vi "DjtgPutTmsTdiBits.vi"(6 "Receive Buffer Size (Bytes)":i32=10, 7 "Overlap?":bool, 8 "Error In":errorcluster, 9 "Num Bit Pairs":u32, 10 "Data To Send":u8[](array[numeric]), 11 "Device Number":u32) -> (0 "Error Out":errorcluster, 2 "Data":u8[](array[numeric]), 3 "Device Number":u32)   [LabVIEW 2011, in "LVH-Adept.lvlib" / "DJTG.lvlib"]
doc: "Regardless of the scan format configuration, the rgbSnd parameter specifies a buffer containing the sequence of the TDI and TMS bits that should be shifted. The TDI bits contained in rgbSnd are automatically complemented as necessary. For example, if the current scan format is OScan1 and rgbSnd[0] = 0xAB and rgbSnd[1] = 0xEB then first byte of TDI bits is 0x91 and 0x6E will be shifted for the nTDI bits. For more information regarding the format of the data shifted by this function, see the section titled “Scan Formats.”"
uses:
  DJTG.lvlib
  Private/Type Defs/Error.ctl
  Resources/djtg.dll
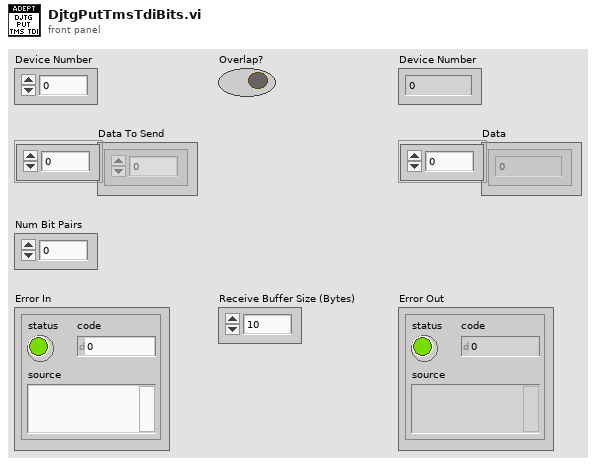
[diagram p1: front panel]
types:
  T1 = typedef "LVH-Adept.lvlib/DJTG.lvlib/Error.ctl" = enum16{"Unknown", "Enable", "PutTmsTdiBits", "GetTdoBits", "Disable", "Close", "Set Aux Reset", "Port Properties", "Get Speed", "Set Speed", "Get Port Count", "Get Batch Properties", "Enable Port", "Set Tmd Tdi Tck", "Get Tms Tdi Tdo Tck", "Put Tdi Bits", "Put Tms Bits", "Clock Tck", "Wait", "Batch"}
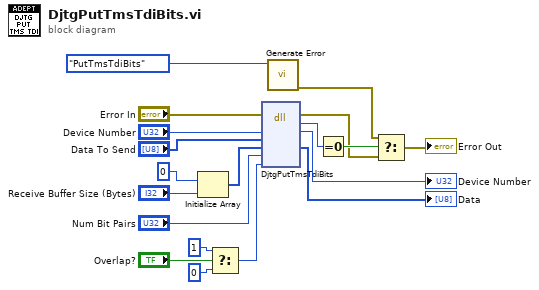
[diagram p0: block diagram]
diagram:
  n1 = Initialize Array(u8 0, "Receive Buffer Size (Bytes)") -> (w1:u8[])
  n2 = Select(t=u8 1, s="Overlap?", f=u8 0) -> (s? t:f=w5:u8)
  n3 = dll-call lib="C:/github/labviewhacker/LVH-Adept/LabVIEW/vi.lib/LabVIEW Hacker/Adept/Private/Resources/djtg.dll" fn="DjtgPutTmsTdiBits"(error in="Error In", "HIF"="Device Number", "rgbSnd"="Data To Send", "rgbRcv"=w1, "cbitpairs"="Num Bit Pairs", "fOverlap"=w5) -> (error out=w15:errorcluster, "Success"=w17:u32, "HIF"=→"Device Number":u32, "rgbRcv"=→"Data":u8[])  [unwired: 5 in, 1 out]
  n4 = call "Generate Error.vi"("DJTG Error"=Error."PutTmsTdiBits") -> ("Error Out"=w16:errorcluster)  [unwired: 10 in]
  n5 = Equal To 0?(x=w17) -> (x = 0?=w18:bool)
  n6 = Select(t=w16, s=w18, f=w15) -> (s? t:f=→"Error Out":errorcluster)
